vi "TTiPS.vi"(11 "VISA Refnum in":refnum<visa-resource-name>) -> (3 "TTi PS actual voltage":string)   [LabVIEW 2019]
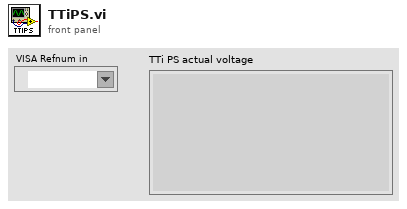
[diagram p1: front panel]
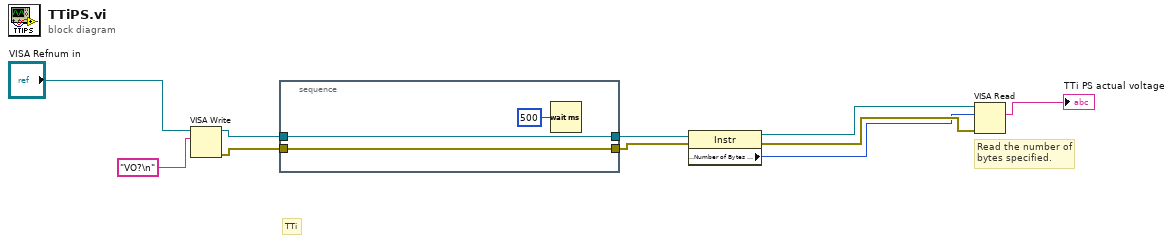
[diagram p0: block diagram]
diagram:
  # "TTi"
  # "Read the number of bytes specified."
  n1 = VISA Write(VISA resource name="VISA Refnum in", write buffer="VO?\n") -> (VISA resource name out=w9:refnum<visa-resource-name>, error out=w10:errorcluster)  [unwired: 1 in, 1 out]
  n2 = stacked-sequence {
    tunnel: w10 -> [w13]
    tunnel: [w13] -> w2
    tunnel: w9 -> [w12]
    tunnel: [w12] -> w3
    frame #0 {
      n3 = Wait (ms)(milliseconds to wait=u32 500) -> ()  [unwired: 1 out]
    }
  }
  n4 = property class="Instr"(reference=w3, error in=w2) -> (reference out=w8:refnum<visa-resource-name>, error out=w7:errorcluster, "Serial Settings:Number of Bytes at Serial Port"=w6:u32)
  n5 = VISA Read(VISA resource name=w8, byte count=w6, error in (no error)=w7) -> (read buffer=→"TTi PS actual voltage":string)  [unwired: 3 out]
